vi "Kalman filter - P array 1st (SubVI).vi"(1 "P Array In":dbl[][](array[numeric]), 2 "dt":dbl, 3 "Q_Angle":dbl, 4 "Q_Bias":dbl) -> (0 "P Array out":dbl[][](array[numeric]))   [LabVIEW 2013]
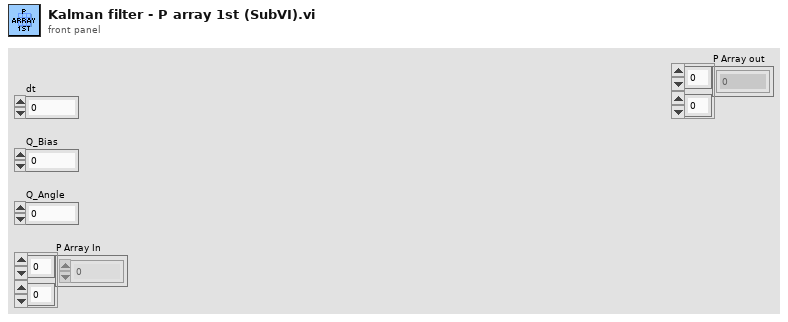
[diagram p1: front panel]
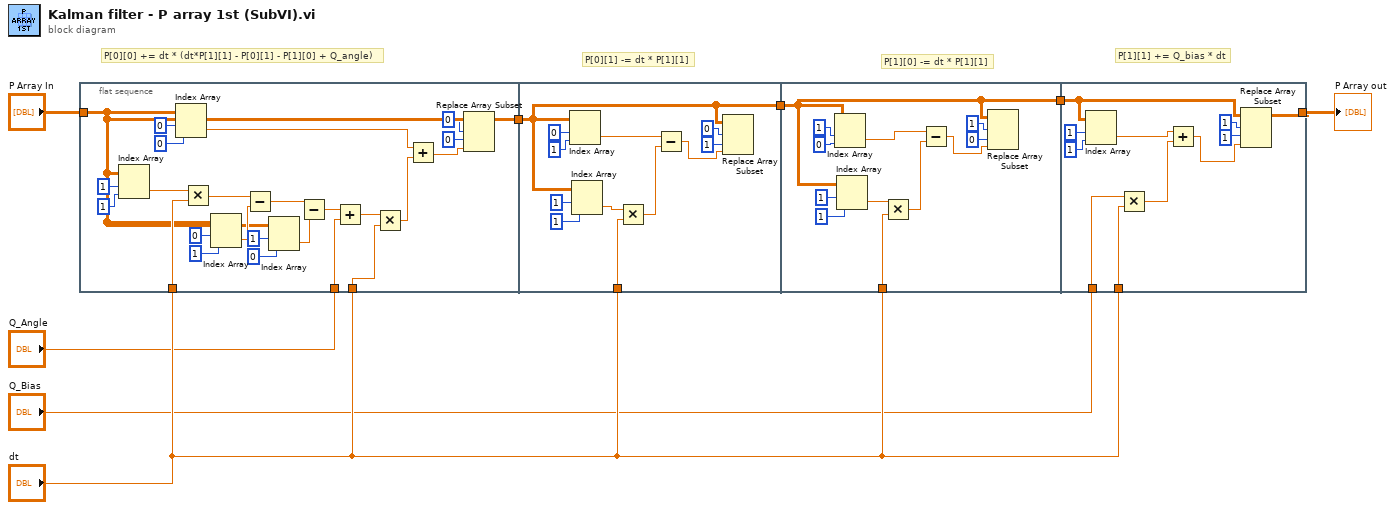
[diagram p0: block diagram]
diagram:
  # "P[1][1] += Q_bias * dt"
  # "P[1][0] -= dt * P[1][1]"
  # "P[0][1] -= dt * P[1][1]"
  # "P[0][0] += dt * (dt*P[1][1] - P[0][1] - P[1][0] + Q_angle)"
  n1 = flat-sequence {
    tunnel: "P Array In" -> [w13]
    tunnel: "Q_Angle" -> [w19]
    tunnel: "dt" -> [w14]
    tunnel: "dt" -> [w15]
    tunnel: [w9] -> w8
    tunnel: w8 -> [w34]
    tunnel: "dt" -> [w39]
    tunnel: [w34] -> w7
    tunnel: w7 -> [w46]
    tunnel: "dt" -> [w47]
    tunnel: [w46] -> w6
    tunnel: w6 -> [w59]
    tunnel: "Q_Bias" -> [w65]
    tunnel: "dt" -> [w64]
    tunnel: [w58] -> w1
    frame #0 {
      n2 = Index Array(array=w13, index (row)=1, index (col)=1) -> (element=w29:dbl)
      n3 = Index Array(array=w13, index (row)=0, index (col)=0 ("disabled index (col)")) -> (element=w16:dbl)
      n4 = Multiply(x=w29, y=w14) -> (x*y=w28:dbl)
      n5 = Index Array(array=w13, index (row)=0, index (col)=1) -> (element=w25:dbl)
      n6 = Subtract(x=w28, y=w25) -> (x-y=w24:dbl)
      n7 = Index Array(array=w13, index (row)=1, index (col)=0) -> (element=w21:dbl)
      n8 = Subtract(x=w24, y=w21) -> (x-y=w20:dbl)
      n9 = Add(x=w20, y=w19) -> (x+y=w18:dbl)
      n10 = Multiply(x=w18, y=w15) -> (x*y=w17:dbl)
      n11 = Add(x=w16, y=w17) -> (x+y=w10:dbl)
      n12 = Replace Array Subset(array=w13, new element=w10, index (row)=0, index (col)=0 ("disabled index (col)")) -> (w9:dbl[][])
    }
    frame #1 {
      n13 = Index Array(array=w34, index (row)=0, index (col)=1 ("disabled index (col)")) -> (element=w43:dbl)
      n14 = Index Array(array=w34, index (row)=1, index (col)=1) -> (element=w40:dbl)
      n15 = Multiply(x=w40, y=w39) -> (x*y=w38:dbl)
      n16 = Subtract(x=w43, y=w38) -> (x-y=w35:dbl)
      n17 = Replace Array Subset(array=w34, new element=w35, index (row)=0, index (col)=1) -> ()  [unwired: 1 out]
    }
    frame #2 {
      n18 = Index Array(array=w46, index (row)=1, index (col)=0 ("disabled index (col)")) -> (element=w55:dbl)
      n19 = Index Array(array=w46, index (row)=1, index (col)=1) -> (element=w52:dbl)
      n20 = Multiply(x=w52, y=w47) -> (x*y=w51:dbl)
      n21 = Subtract(x=w55, y=w51) -> (x-y=w48:dbl)
      n22 = Replace Array Subset(array=w46, new element=w48, index (row)=1, index (col)=0) -> ()  [unwired: 1 out]
    }
    frame #3 {
      n23 = Index Array(array=w59, index (row)=1, index (col)=1 ("disabled index (col)")) -> (element=w66:dbl)
      n24 = Multiply(x=w65, y=w64) -> (x*y=w63:dbl)
      n25 = Add(x=w66, y=w63) -> (x+y=w60:dbl)
      n26 = Replace Array Subset(array=w59, new element=w60, index (row)=1, index (col)=1) -> (w58:dbl[][])
    }
  }
  "P Array out" <- w1
